vi "Filter Set Averaging Frame Count.vi"(8 "error in (no error)":errorcluster, 11 "frames":i32) -> (0 "error out":errorcluster, 3 "function return":u32)   [LabVIEW 2014, in "atmcd32d.lvlib"]
doc: "unsigned int WINAPI Filter_SetAveragingFrameCount(int frames);"
uses:
  atmcd32d.lvlib
  atmcd32d.dll
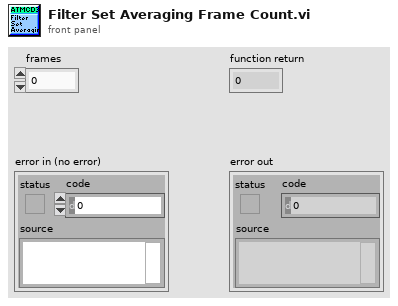
[diagram p1: front panel]
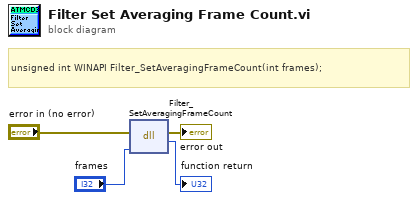
[diagram p0: block diagram]
diagram:
  # "unsigned int WINAPI Filter_SetAveragingFrameCount(int frames);"
  n1 = dll-call lib="C:/Users/Bakir/Documents/Lambda2-Testing/lib/Andorlib/atmcd32d.*" fn="Filter_SetAveragingFrameCount"(error in="error in (no error)", "frames"="frames") -> (error out=→"error out":errorcluster, →"function return":u32)  [unwired: 3 in, 1 out]
